vi "Enable BC.vi"(7 "Virtual Memory Unit in":refnum<class "Virtual Memory Unit.lvclass">, 8 "error in (no error)":errorcluster, 11 "Bus Controller in":refnum<class "Bus Controller.lvclass">) -> (0 "error out":errorcluster, 3 "Bus Controller out":refnum<class "Bus Controller.lvclass">, 5 "Virtual Memory Unit out":refnum<class "Virtual Memory Unit.lvclass">)   [LabVIEW 2020, in "BCI-1553 API.lvlib" / "Bus Controller.lvclass"]
doc: "Enables the operation of this Bus Controller."
uses:
  Bus Controller.lvclass
  Dependencies/Virtual Memory Unit/Virtual Memory Unit.lvclass
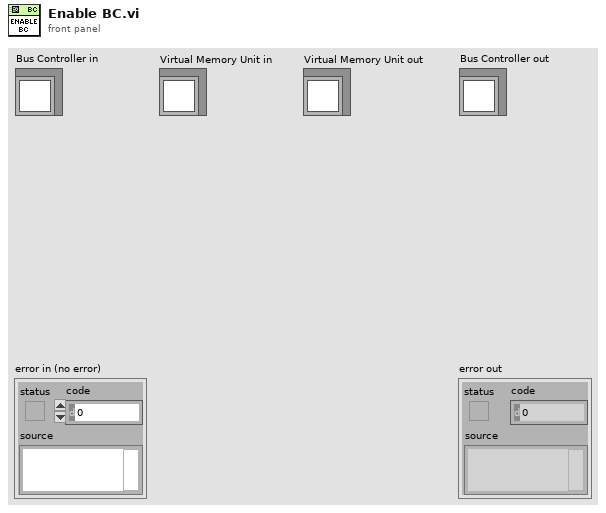
[diagram p1: front panel]
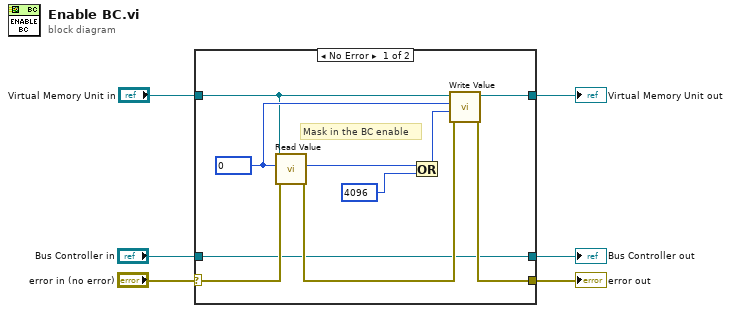
[diagram p0: block diagram]
diagram:
  n1 = case shown="No Error" "error in (no error)" {
    selector: "error in (no error)" -> [w13 w19]
    tunnel: [w11 w19] -> w3
    tunnel: [w10 w18] -> w4
    tunnel: "Bus Controller in" -> [w10 w18]
    tunnel: "Virtual Memory Unit in" -> [w9 w17]
    tunnel: [w8 w17] -> w1
    frame No Error {
      w14 = 0 ("Address")
      # "Mask in the BC enable"
      n2 = call "Read Value.vi"("error in (no error)"=w13, "Index"=w14, "Virtual Memory Unit in"=w9) -> ("error out"=w12:errorcluster, "Value"=w16:u16)  [unwired: 7 in]
      n3 = Or(x=w16, y=u16 4096 ("Address")) -> (x .or. y?=w15:u16)
      n4 = call "Write Value.vi"("error in (no error)"=w12, "Value"=w15, "Index"=w14, "Virtual Memory Unit in"=w9) -> ("error out"=w11:errorcluster, "Virtual Memory Unit out"=w8:refnum<class "Virtual Memory Unit.lvclass">)  [unwired: 6 in]
    }
    frame Error {
    }
  }
  "error out" <- w3
  "Bus Controller out" <- w4
  "Virtual Memory Unit out" <- w1
